vi "Before After View.vi"(10 "after":T1[](array[typedef]) {"height" format="%+4.3f"; "pixel_y" format="%+4.3f"; "pixel_x" format="%+4.3f"; "orientation" format="%+4.3f"; "y" format="%+4.3f"; "confidence" format="%4.3f"; "x" format="%+4.3f"}, 11 "before":T1[](array[typedef]) {"height" format="%+4.3f"; "pixel_y" format="%+4.3f"; "pixel_x" format="%+4.3f"; "orientation" format="%+4.3f"; "y" format="%+4.3f"; "confidence" format="%4.3f"; "x" format="%+4.3f"}) -> ()   [LabVIEW 2017]
uses:
  <vilib>/Analysis/Matrix/Datatypes/RealMatrix.ctl
  <vilib>/Analysis/Matrix/NI_Matrix.lvlib
  SSL Detection Robot.ctl
panel:
  out "Waveform Chart":sgl[][](graph)
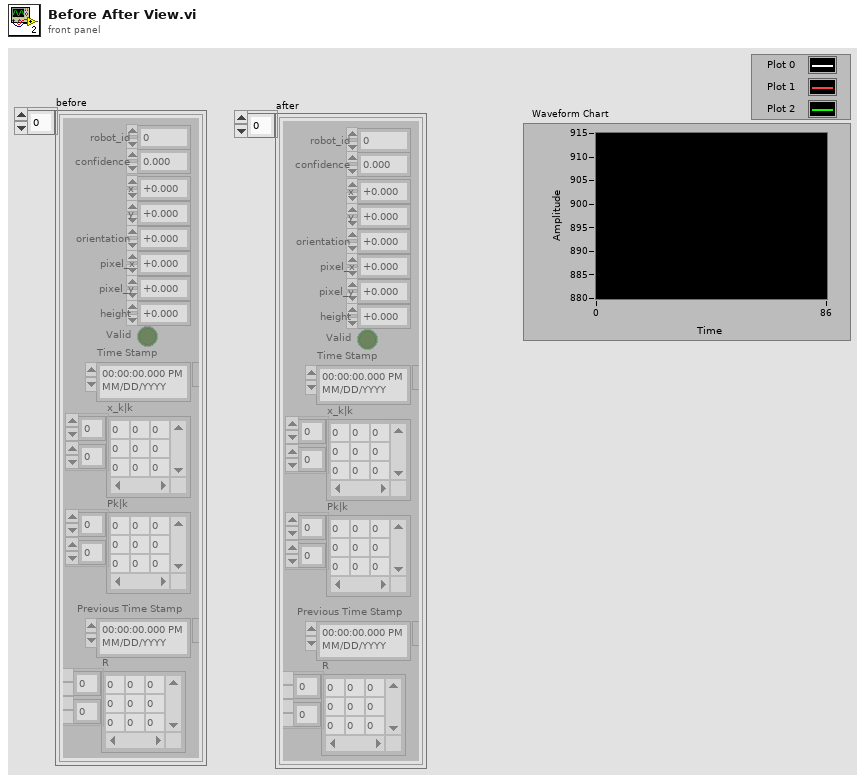
[diagram p1: front panel]
types:
  T1 = typedef "SSL Detection Robot.ctl" = cluster{"x":sgl, "robot_id":u32, "confidence":sgl, "y":sgl, "orientation":sgl, "pixel_x":sgl, "pixel_y":sgl, "height":sgl, "Valid":bool, "Time Stamp":timestamp, "x_k|k":T2, "Pk|k":T2, "Previous Time Stamp":timestamp, "R":T2}
  T2 = typedef "NI_Matrix.lvlib/RealMatrix.ctl" = dbl[][]
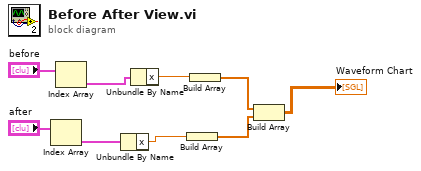
[diagram p0: block diagram]
diagram:
  n1 = Index Array(array="after") -> (element=w6:T1)  [unwired: 1 in]
  n2 = Index Array(array="before") -> (element=w7:T1)  [unwired: 1 in]
  n3 = Unbundle By Name(w6) -> ("x"=w5:sgl)
  n4 = Unbundle By Name(w7) -> ("x"=w1:sgl)
  n5 = Build Array(w5) -> (w3:sgl[])
  n6 = Build Array(w1) -> (w4:sgl[])
  n7 = Build Array(w4, w3) -> (→"Waveform Chart":sgl[][])
